vi "log测试.vi"() -> ()   [LabVIEW 2019, in "test.lvlib"]
uses:
  SubVI/test.lvlib
  <vilib>/Utility/file.llb/Write Delimited Spreadsheet (DBL).vi
panel:
  out "添加的数组":dbl[](array[numeric])
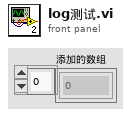
[diagram p1: front panel]
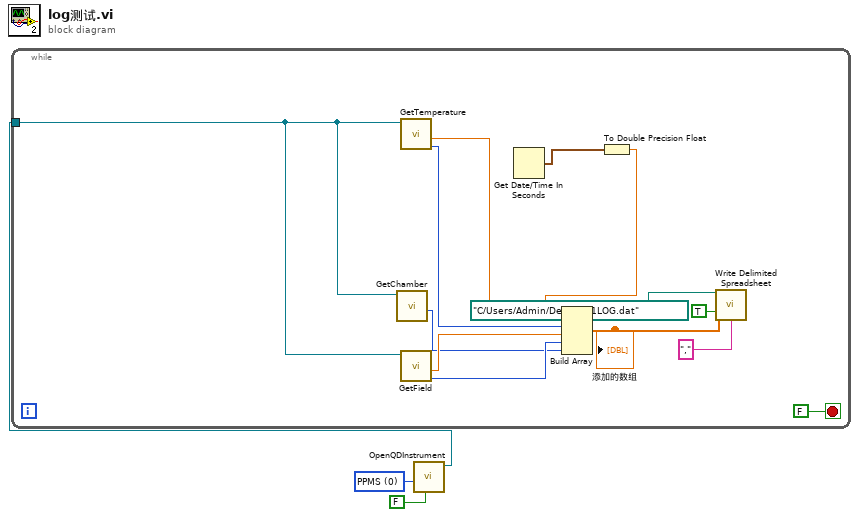
[diagram p0: block diagram]
diagram:
  w3 = 0 items=["PPMS", "VersaLab", "DynaCool", "SVSM"] ("Instrument Type")
  n1 = call "OpenQDInstrument.vi"("Remote"=FALSE, "Instrument Type"=w3) -> ("Instrument Ref"=w2:refnum<k24>)  [unwired: 6 in, 1 out]
  n2 = while {
    tunnel: w2 -> [w16]
    stop <- FALSE stop-if-true
    n3 = call "GetChamber.vi"("Instrument Ref In"=w16) -> ("Chamber\nStatus"=w9:i32)  [unwired: 3 in, 3 out]
    n4 = call "GetTemperature.vi"("Instrument Ref In"=w16) -> ("Temperature\nStatus"=w13:i32, "Temperature"=w14:dbl)  [unwired: 4 in, 3 out]
    n5 = call "GetField.vi"("Instrument Ref In"=w16) -> ("Field\nStatus"=w11:i32, "Field"=w12:dbl)  [unwired: 4 in, 3 out]
    n6 = Get Date/Time In Seconds() -> (seconds since 1Jan1904=w15:timestamp)
    n7 = To Double Precision Float(number=w15) -> (double precision float=w10:dbl)
    n8 = Build Array(w10, w14, w13, w12, w11, w9) -> (w8:dbl[])
    "添加的数组" <- w8
    n9 = call-poly <vilib>:"Write Delimited Spreadsheet.vi"("file path (dialog if empty)"=path "C:/Users/Admin/Desktop/1LOG.dat", "1D data"=w8, "append to file? (new file:F)"=TRUE, "delimiter (\\t)"="," ("delimiter (\\t)")) -> ()  [unwired: 10 in, 2 out]
  }
